vi "ti2_setEnableJoystick.vi"(8 "error in (no error)":errorcluster, 11 "value":bool) -> (0 "error out":errorcluster)   [LabVIEW 2023, in "ti2lv.lvlib"]
uses:
  ti2lv.lvlib
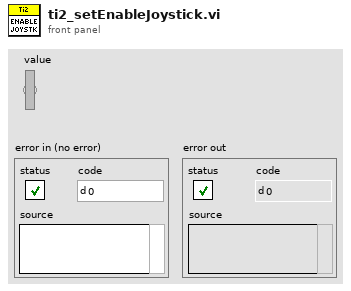
[diagram p1: front panel]
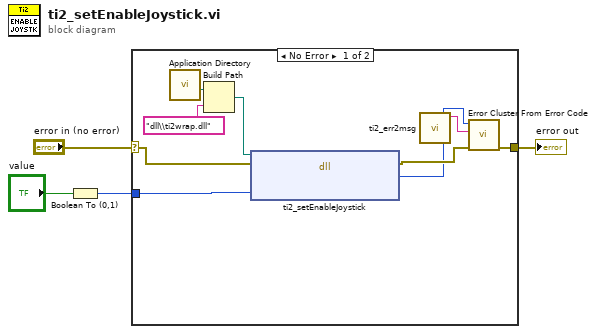
[diagram p0: block diagram]
diagram:
  n1 = Boolean To (0,1)(Boolean="value") -> (0, 1=w2:i16)
  n2 = case shown="No Error" "error in (no error)" {
    selector: "error in (no error)" -> [w10 w14]
    tunnel: [w13 w14] -> w4
    tunnel: w2 -> [w11 _]
    frame No Error {
      n3 = call <vilib>:"Application Directory.vi"() -> ("Application Directory"=w6:path)
      n4 = Build Path(base path=w6, name or relative path="dll\\ti2wrap.dll") -> (appended path=w5:path)
      n5 = dll-call lib="?" fn="ti2_setEnableJoystick"(path in=w5, error in=w10, "data"=w11) -> (error out=w9:errorcluster, "return type"=w8:i32)  [unwired: 2 in, 1 out]
      n6 = call "ti2_err2msg.vi"("Error Code"=w8) -> ("Error Message"=w12:string)  [unwired: 10 in]
      n7 = call <vilib>:"Error Cluster From Error Code.vi"("error in (no error)"=w9, "error message (\"\")"=w12, "error code (0)"=w8) -> ("error out"=w13:errorcluster)  [unwired: 6 in]
    }
    frame Error {
    }
  }
  "error out" <- w4
